vi "JT_ueberwachung.vi"(8 "Warning In":string, 11 "System Monitor Variables":T1={"Time"=array[65275 elements], "LI1CH1"=array[65275 elements], "LI1CH2"=array[65275 elements], "LI2CH1"=array[65275 elements], "LI2CH2"=array[65275 elements], "LI3CH1"=[], "LI3CH2"=[], "Field"=array[65275 elements], "N_Level"=array[65275 elements], "H_Level"=array[65275 elements], "Heat_370"=array[65275 elements], "Sorb_Heat"=array[65275 elements], "Still_Heat"=array[65275 elements], "Capacity"=array[65275 elements], "Loss"=array[65275 elements], "Magnet_Temperature"=array[65275 elements], "Lam_Pressure"=array[65275 elements], "Lam_NValve"=array[65275 elements], "370-T1"=array[65275 elements], "370-T2"=array[65275 elements], "370-T3"=array[65275 elements], "370-T4"=array[65275 elements], "370-T5"=array[65275 elements], "370-R1"=array[65275 elements], "370-R2"=array[65275 elements], "370-R3"=array[65275 elements], "370-R4"=array[65275 elements], "370-R5"=array[65275 elements], "372-T1"=array[65275 elements], "372-T2"=array[65275 elements], "372-T3"=array[65275 elements], "372-T4"=array[65275 elements], "372-T5"=array[65275 elements], "372-T6"=[], "372-R1"=array[65275 elements], "372-R2"=array[65275 elements], "372-R3"=array[65275 elements], "372-R4"=array[65275 elements], "372-R5"=array[65275 elements], "372-R6"=[], "Nada"=[nan], "K2440_Res"=array[65275 elements], "K2440_Current"=array[65275 elements], "VTI_Heater"=array[65275 elements], "VTI_NValve"=array[65275 elements], "LS340_Heater"=[], "K6221_Amplitude"=array[65275 elements], "K6221_Frequency"=array[65275 elements], "Cond_Pressure"=array[65275 elements], "Still_Pressure"=array[65275 elements], "FP_Out_Pressure"=array[65275 elements], "Dump_Pressure"=array[65275 elements], "V1"=array[65275 elements], "V2"=array[65275 elements], "V4"=array[65275 elements], "V5"=array[65275 elements], "V9"=array[65275 elements], "Forepump"=array[65275 elements], "Compressor"=array[65275 elements], "K6221_Offset"=array[65275 elements], "BoxTemp"=[], "By"=[], "Bz"=[], "Phi"=[], "heater-recond (%)"=[], "Dewar Pressure "=[], "JT-SP-Control"=[], "350 T1"=[], "350 T2"=[], "350 T3"=[], "350 T4"=[], "350 R1"=[], "350 R2"=[], "350 R3"=[], "350 R4"=[], "Angle"=[], "VTI CH1"=array[65275 elements], "VTI CH2"=array[65275 elements], "VTI CH3"=array[65275 elements], "ColdTrap"=[], "Mischer Pot"=[], "G1 (mbar)"=[], "G3 (mbar) "=[], "G4 (mbar)"=[], "IVC (mbar)"=[], "P2 (mbar) "=[], "Pot mischer (mbar)"=[], "AVS Control Channel (K)"=[], "AVS Control Channel (RES)"=[], "AVS  Channel 5 (RES) "=[], "LI3CH3"=[], "LI3CH4"=[], "LI1CH3"=[], "LI1CH4"=[], "LI2CH3"=[], "LI2CH4"=[], "Volt"=[], "Watt"=[], "Torque Angle"=[], "Dewar heater (W)"=[], "PSU Voltage"=[], "Turbopump"=[], "372-R7"=[], "372-T7"=[], "SIM921 Ch1"=[], " He3 Temp1"=[], " He3 Temp 2"=[], "LI4CH1"=[], "LI4CH2"=[], "372-T8"=[], "372-R8"=[]}) -> (0 "Warning-Bool":bool=TRUE, 3 "Warning Out":string)   [LabVIEW 2019]
uses:
  Global/Global Variables/System Monitor Cluster.ctl
panel:
  out "Warning-Bool":bool
  out "Warning":string
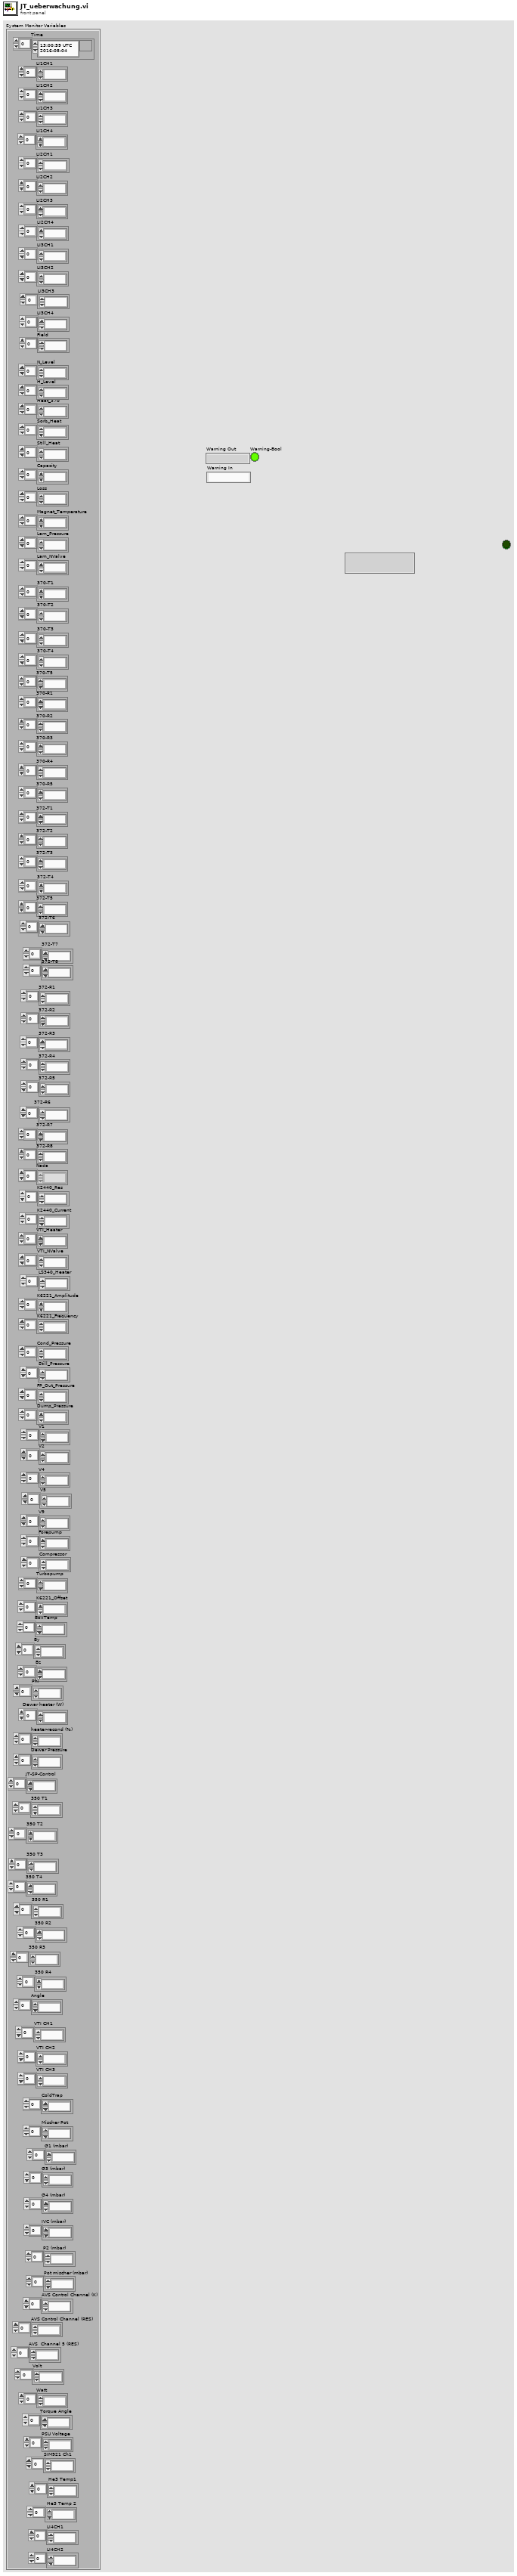
[diagram p1: front panel]
types:
  T1 = typedef "System Monitor Cluster.ctl" = cluster{"Time":timestamp[], "LI1CH1":dbl[], "LI1CH2":dbl[], "LI2CH1":dbl[], "LI2CH2":dbl[], "LI3CH1":dbl[], "LI3CH2":dbl[], "Field":dbl[], "N_Level":dbl[], "H_Level":dbl[], "Heat_370":dbl[], "Sorb_Heat":dbl[], "Still_Heat":dbl[], "Capacity":dbl[], "Loss":dbl[], "Magnet_Temperature":dbl[], "Lam_Pressure":dbl[], "Lam_NValve":dbl[], "370-T1":dbl[], "370-T2":dbl[], "370-T3":dbl[], "370-T4":dbl[], "370-T5":dbl[], "370-R1":dbl[], "370-R2":dbl[], "370-R3":dbl[], "370-R4":dbl[], "370-R5":dbl[], "372-T1":dbl[], "372-T2":dbl[], "372-T3":dbl[], "372-T4":dbl[], "372-T5":dbl[], "372-T6":dbl[], "372-R1":dbl[], "372-R2":dbl[], "372-R3":dbl[], "372-R4":dbl[], "372-R5":dbl[], "372-R6":dbl[], "Nada":dbl[], "K2440_Res":dbl[], "K2440_Current":dbl[], "VTI_Heater":dbl[], "VTI_NValve":dbl[], "LS340_Heater":dbl[], "K6221_Amplitude":dbl[], "K6221_Frequency":dbl[], "Cond_Pressure":dbl[], "Still_Pressure":dbl[], "FP_Out_Pressure":dbl[], "Dump_Pressure":dbl[], "V1":dbl[], "V2":dbl[], "V4":dbl[], "V5":dbl[], "V9":dbl[], "Forepump":dbl[], "Compressor":dbl[], "K6221_Offset":dbl[], "BoxTemp":dbl[], "By":dbl[], "Bz":dbl[], "Phi":dbl[], "heater-recond (%)":dbl[], "Dewar Pressure ":dbl[], "JT-SP-Control":dbl[], "350 T1":dbl[], "350 T2":dbl[], "350 T3":dbl[], "350 T4":dbl[], "350 R1":dbl[], "350 R2":dbl[], "350 R3":dbl[], "350 R4":dbl[], "Angle":dbl[], "VTI CH1":dbl[], "VTI CH2":dbl[], "VTI CH3":dbl[], "ColdTrap":dbl[], "Mischer Pot":dbl[], "G1 (mbar)":dbl[], "G3 (mbar) ":dbl[], "G4 (mbar)":dbl[], "IVC (mbar)":dbl[], "P2 (mbar) ":dbl[], "Pot mischer (mbar)":dbl[], "AVS Control Channel (K)":dbl[], "AVS Control Channel (RES)":dbl[], "AVS  Channel 5 (RES) ":dbl[], "LI3CH3":dbl[], "LI3CH4":dbl[], "LI1CH3":dbl[], "LI1CH4":dbl[], "LI2CH3":dbl[], "LI2CH4":dbl[], "Volt":dbl[], "Watt":dbl[], "Torque Angle":dbl[], "Dewar heater (W)":dbl[], "PSU Voltage":dbl[], "Turbopump":dbl[], "372-R7":dbl[], "372-T7":dbl[], "SIM921 Ch1":dbl[], " He3 Temp1":dbl[], " He3 Temp 2":dbl[], "LI4CH1":dbl[], "LI4CH2":dbl[], "372-T8":dbl[], "372-R8":dbl[]}
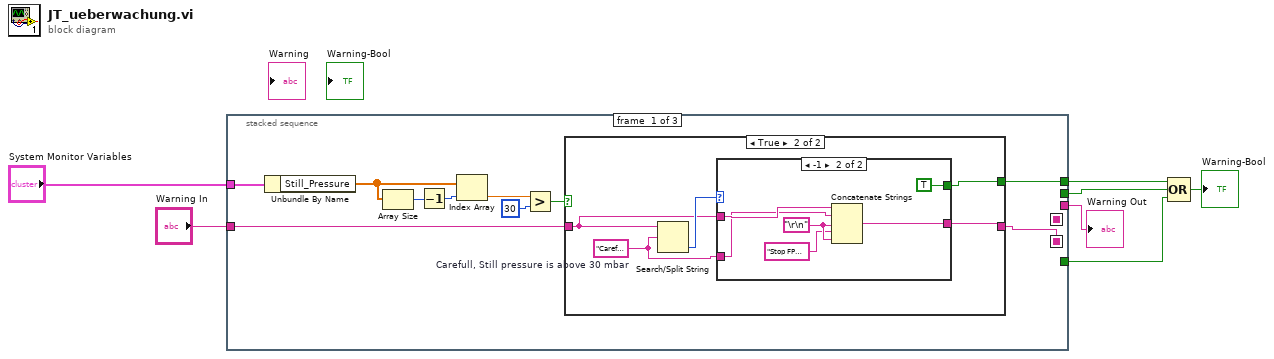
[diagram p0: block diagram]
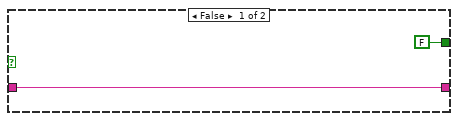
[diagram p2: hidden frame]
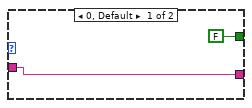
[diagram p3: hidden frame]
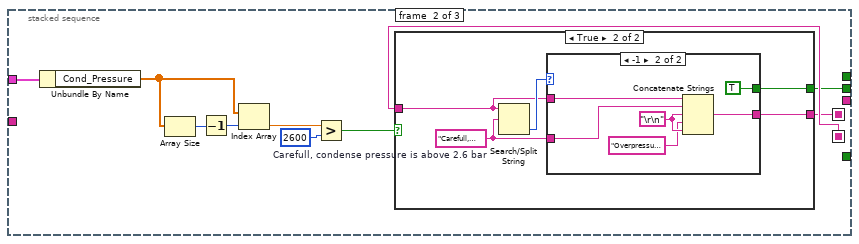
[diagram p4: hidden frame]
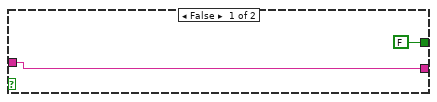
[diagram p5: hidden frame]
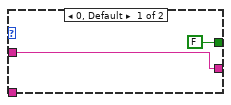
[diagram p6: hidden frame]
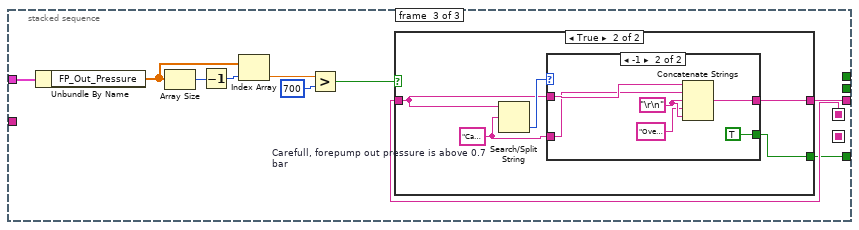
[diagram p7: hidden frame]
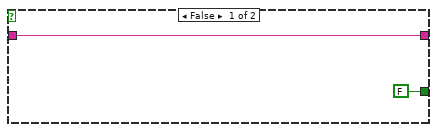
[diagram p8: hidden frame]
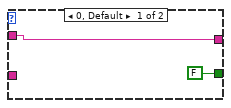
[diagram p9: hidden frame]
diagram:
  n1 = stacked-sequence {
    seq-local: [w12 _ _] -> [_ w36 _]
    seq-local: [_ w34 _] -> [_ _ w60]
    tunnel: "System Monitor Variables" -> [w17 w35 w61]
    tunnel: "Warning In" -> [w9 _ _]
    tunnel: [_ _ w59] -> w5
    tunnel: [_ _ w58] -> w2
    tunnel: [_ w33 _] -> w3
    tunnel: [w8 _ _] -> w4
    frame #0 {
      n2 = Unbundle By Name(w17) -> ("Still_Pressure"=w13:dbl[])
      n3 = Array Size(array=w13) -> (size(s)=w11:i32)
      n4 = Decrement(x=w11) -> (x-1=w10:i32)
      n5 = Index Array(array=w13, index=w10) -> (element=w14:dbl)
      n6 = Greater?(x=w14, y=30) -> (0:w15:bool)
      n7 = case shown="True" w15 {
        tunnel: [w18 w21] -> w12
        tunnel: w9 -> [w18 w22]
        tunnel: [FALSE w20] -> w8
        frame False {
        }
        frame True {
          w23 = "Carefull, Still pressure is above 30 mbar "  # Carefull, Still pressure is above 30 mbar
          n8 = Search/Split String(string=w22, search string/char (-)=w23) -> (offset of match=w24:i32)  [unwired: 1 in, 2 out]
          n9 = case shown="-1" w24 {
            tunnel: w23 -> [_ w29]
            tunnel: w22 -> [w25 w30]
            tunnel: [w25 w28] -> w21
            tunnel: [FALSE TRUE] -> w20
            frame 0, Default {
            }
            frame -1 {
              w32 = "\r\n"
              n10 = Concatenate Strings(w30, w29, w32, "Stop FP immediatelly and open V9 to prevent overpressure", w32) -> (w28:string)
            }
          }
        }
      }
    }
    frame #1 {
      n11 = Unbundle By Name(w35) -> ("Cond_Pressure"=w39:dbl[])
      n12 = Array Size(array=w39) -> (size(s)=w38:i32)
      n13 = Decrement(x=w38) -> (x-1=w37:i32)
      n14 = Index Array(array=w39, index=w37) -> (element=w40:dbl)
      n15 = Greater?(x=w40, y=2600) -> (0:w41:bool)
      n16 = case shown="True" w41 {
        tunnel: [w43 w46] -> w34
        tunnel: w36 -> [w43 w47]
        tunnel: [FALSE w45] -> w33
        frame False {
        }
        frame True {
          w48 = "Carefull, condense pressure is above 2.6 bar "  # Carefull, condense pressure is above 2.6 bar
          n17 = Search/Split String(string=w47, search string/char (-)=w48) -> (offset of match=w49:i32)  [unwired: 1 in, 2 out]
          n18 = case shown="-1" w49 {
            tunnel: w48 -> [_ w54]
            tunnel: w47 -> [w50 w55]
            tunnel: [w50 w53] -> w46
            tunnel: [FALSE TRUE] -> w45
            frame 0, Default {
            }
            frame -1 {
              w57 = "\r\n"
              n19 = Concatenate Strings(w55, w54, w57, "Overpressure Valve will open any second. Reduce condensor inlet pressure, Close V9", w57) -> (w53:string)
            }
          }
        }
      }
    }
    frame #2 {
      n20 = Unbundle By Name(w61) -> ("FP_Out_Pressure"=w64:dbl[])
      n21 = Array Size(array=w64) -> (size(s)=w63:i32)
      n22 = Decrement(x=w63) -> (x-1=w62:i32)
      n23 = Index Array(array=w64, index=w62) -> (element=w65:dbl)
      n24 = Greater?(x=w65, y=700) -> (0:w66:bool)
      n25 = case shown="True" w66 {
        tunnel: [w68 w71] -> w59
        tunnel: w60 -> [w68 w72]
        tunnel: [FALSE w70] -> w58
        frame False {
        }
        frame True {
          w73 = "Carefull, forepump out pressure is above 0.7 bar "  # Carefull, forepump out pressure is above 0.7 bar
          n26 = Search/Split String(string=w72, search string/char (-)=w73) -> (offset of match=w74:i32)  [unwired: 1 in, 2 out]
          n27 = case shown="-1" w74 {
            tunnel: w73 -> [_ w79]
            tunnel: w72 -> [w75 w80]
            tunnel: [w75 w78] -> w71
            tunnel: [FALSE TRUE] -> w70
            frame 0, Default {
            }
            frame -1 {
              w82 = "\r\n"
              n28 = Concatenate Strings(w80, w79, w82, "Overpressure Valve will open any second. Reduce still pressure. Close V9", w82) -> (w78:string)
            }
          }
        }
      }
    }
  }
  "Warning Out" <- w5
  n29 = Compound Arithmetic op=OR(w4, w3, w2) -> (→"Warning-Bool":bool)
